vi "Create Element Output.vi"(0 "Current Max SP":dbl[](array[numeric]), 1 "Current In":dbl[](array[numeric]), 2 "Current Min SP":dbl[](array[numeric]), 3 "Voltage Max SP":dbl[](array[numeric]), 4 "Voltage In":dbl[](array[numeric]), 5 "Voltage Min SP":dbl[](array[numeric]), 6 "Power Max SP":dbl[](array[numeric]), 7 "Power In":dbl[](array[numeric]), 8 "Error ACT":bool, 9 "Power Min SP":dbl[](array[numeric]), 10 "OnOff ACT":bool, 11 "Output Enable ACT":bool[](array[boolean]), 13 "Feedback In":bool[](array[boolean])) -> (20 "Current Out":dbl[](array[numeric]), 21 "Voltage Out":dbl[](array[numeric]), 22 "Power Out":dbl[](array[numeric]), 23 "Error Channels":i32[](array[numeric]), 24 "Feedback Out":bool[](array[boolean]))   [LabVIEW 2023]
uses:
  <vilib>/numeric/Random Number (Range) DBL.vi
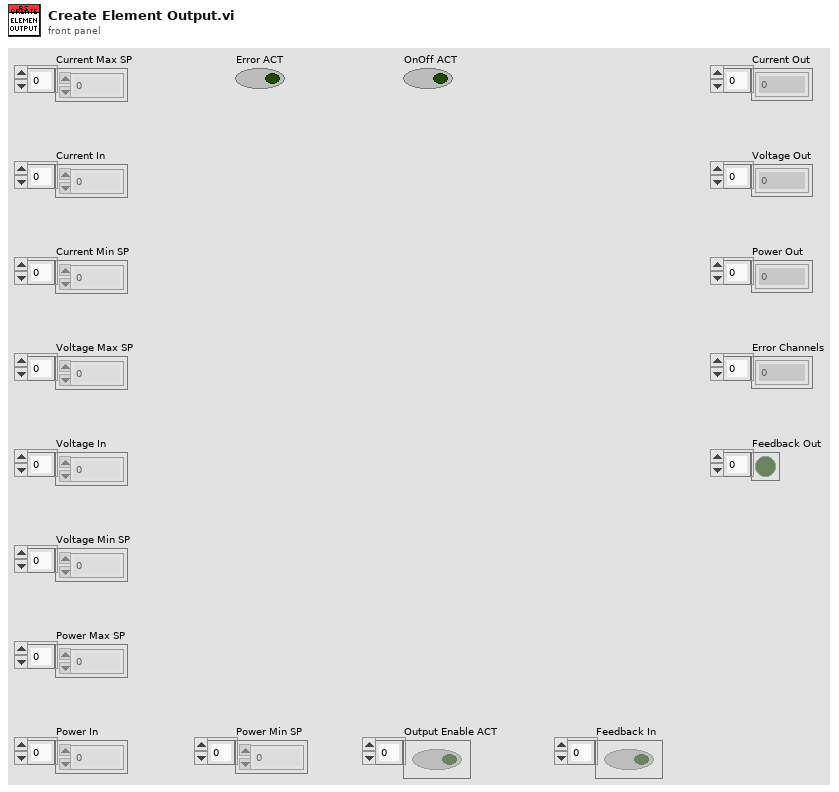
[diagram p1: front panel]
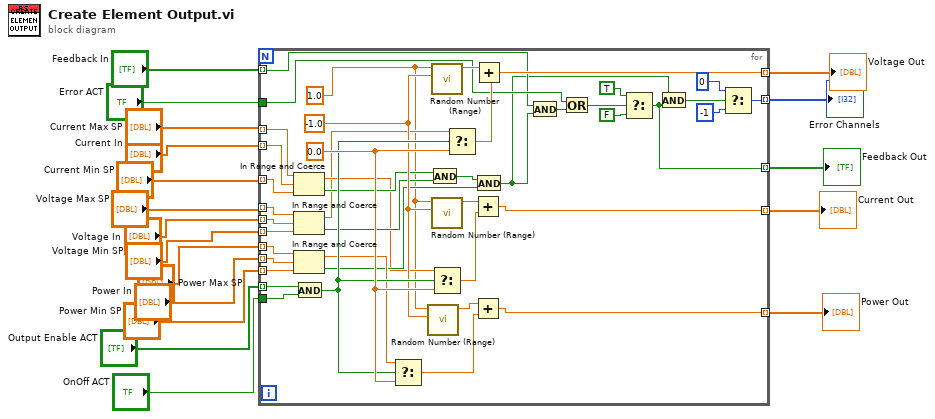
[diagram p0: block diagram]
diagram:
  n1 = for {
    tunnel: "OnOff ACT" -> [w58]
    tunnel: "Output Enable ACT" -> [w59] mode=indexing
    tunnel: "Current In" -> [w61] mode=indexing
    tunnel: "Current Max SP" -> [w60] mode=indexing
    tunnel: [w45] -> w2 mode=indexing
    tunnel: [w42] -> w5 mode=indexing
    tunnel: [w39] -> w1 mode=indexing
    tunnel: "Current Min SP" -> [w55] mode=indexing
    tunnel: "Voltage Max SP" -> [w54] mode=indexing
    tunnel: "Voltage In" -> [w53] mode=indexing
    tunnel: "Voltage Min SP" -> [w52] mode=indexing
    tunnel: "Power Max SP" -> [w50] mode=indexing
    tunnel: "Power Min SP" -> [w49] mode=indexing
    tunnel: "Power In" -> [w48] mode=indexing
    tunnel: "Error ACT" -> [w24]
    tunnel: [w30] -> w4 mode=indexing
    tunnel: [w19] -> w3 mode=indexing
    tunnel: "Feedback In" -> [w23] mode=indexing
    w21 = 1.0 ("upper bound (100)")
    w38 = -1.0 ("lower bound (0)")
    w57 = 0.0 ("f")
    n2 = In Range and Coerce(upper limit=w60, x=w61, lower limit=w55) -> (coerced(x)=w29:dbl, In Range?=w36:bool)
    n3 = In Range and Coerce(upper limit=w54, x=w53, lower limit=w52) -> (coerced(x)=w22:dbl, In Range?=w37:bool)
    n4 = In Range and Coerce(upper limit=w50, x=w48, lower limit=w49) -> (coerced(x)=w51:dbl, In Range?=w35:bool)
    n5 = And(x=w59, y=w58) -> (x .and. y?=w56:bool)
    n6 = Select(t=w51, s=w56, f=w57) -> (s? t:f=w40:dbl)
    n7 = call-poly <vilib>:"Random Number (Range).vi"("lower bound (0)"=w38, "upper bound (100)"=w21) -> ("number"=w41:dbl)  [unwired: 9 in]
    n8 = And(x=w36, y=w37) -> (x .and. y?=w34:bool)
    n9 = call-poly <vilib>:"Random Number (Range).vi"("lower bound (0)"=w38, "upper bound (100)"=w21) -> ("number"=w44:dbl)  [unwired: 9 in]
    n10 = call-poly <vilib>:"Random Number (Range).vi"("lower bound (0)"=w38, "upper bound (100)"=w21) -> ("number"=w47:dbl)  [unwired: 9 in]
    n11 = Select(t=w29, s=w56, f=w57) -> (s? t:f=w46:dbl)
    n12 = Select(t=w22, s=w56, f=w57) -> (s? t:f=w43:dbl)
    n13 = Add(x=w47, y=w46) -> (x+y=w45:dbl)
    n14 = Add(x=w41, y=w40) -> (x+y=w39:dbl)
    n15 = Add(x=w44, y=w43) -> (x+y=w42:dbl)
    n16 = And(x=w34, y=w35) -> (x .and. y?=w20:bool)
    n17 = And(x=w23, y=w20) -> (x .and. y?=w28:bool)
    n18 = Or(x=w24, y=w28) -> (x .or. y?=w27:bool)
    n19 = Select(t=TRUE, s=w27, f=FALSE) -> (s? t:f=w19:bool)
    n20 = And(x=w20, y=w19) -> (x .and. y?=w33:bool)
    n21 = Select(t=0, s=w33, f=-1) -> (s? t:f=w30:i32)
  }
  "Voltage Out" <- w5
  "Error Channels" <- w4
  "Feedback Out" <- w3
  "Current Out" <- w2
  "Power Out" <- w1
